vi "LVLStrHandle.vi"() -> ()   [LabVIEW 2023]
doc: "This function reverses the input string, concatenates it to the original string, and places it in output.\n\nFor information on the data types used for the DLL function, right-click on the Call Library Function node and choose Configure."
uses:
  CLF_Example.dll
panel:
  out "output":string
  in  "input":string="abcd"
  # "Please use alphanumeric characters to get proper results."
  # "See the block diagram for more information."
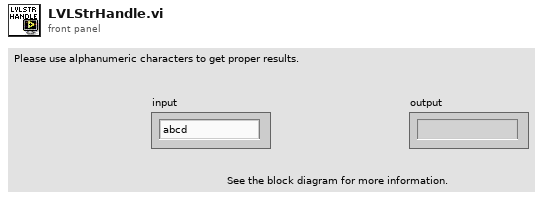
[diagram p1: front panel]
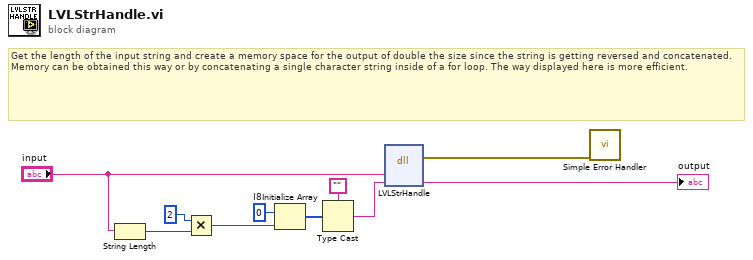
[diagram p0: block diagram]
diagram:
  w9 = i8 0  # I8
  # "Get the length of the input string and create a memory space for the output of double the size since the string is getting reversed and concatenated. Memory can be obtained this way or by concatenating a single character string inside of a for loop. The way displayed here is more efficient."
  n1 = String Length(string="input") -> (length=w4:i32)
  n2 = Multiply(x=2 ("Double"), y=w4) -> (x*y=w3:i32)
  n3 = Initialize Array(w9, w3) -> (w7:i8[])
  n4 = Type Cast(type="", x=w7) -> (*(type *) &x=w5:string)
  n5 = dll-call lib="c:/dev/_r/4/eng/lv-core/lvpostprocessingd/lv_mc_x86_64/dist_i386/examples/Connectivity/Libraries and Executables/DLL Calling VIs/CLF_Example**.*" fn="LVLStrHandle"("input"="input", "output"=w5) -> (error out=w2:errorcluster, "output"=→"output":string)  [unwired: 3 in, 3 out]
  n6 = call <vilib>:"Simple Error Handler.vi"("error in (no error)"=w2) -> ()  [unwired: 4 in, 5 out]
